vi "Fire Update.vi"(8 "error in (no error)":errorcluster, 11 "Recipe Step in":refnum<class "Recipe Step.lvclass">) -> (0 "error out":errorcluster, 3 "Recipe Step out":refnum<class "Recipe Step.lvclass">)   [LabVIEW 2018, in "Temp Recipe.lvlib" / "Recipe Step.lvclass"]
uses:
  Recipe Step.lvclass
  Update Event Data.ctl
  Recipe Step.lvclass/Recipe Step.ctl
  Temp Recipe.lvlib
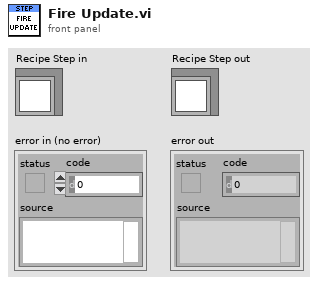
[diagram p1: front panel]
types:
  T1 = typedef "Temp Recipe.lvlib/Update Event Data.ctl" = bool
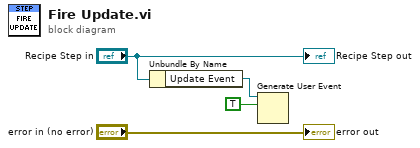
[diagram p0: block diagram]
diagram:
  n1 = Unbundle By Name("Recipe Step in") -> ("Update Event"=w2:refnum<user-event>)
  n2 = Generate User Event(user event=w2, event data cluster=T1 TRUE ("event data")) -> ()  [unwired: 2 in, 2 out]
  "error out" <- "error in (no error)"
  "Recipe Step out" <- "Recipe Step in"
